vi "Get cif_manager_DestroyPluginLoaderResponse.vi"(8 "error in (no error)":errorcluster, 11 "gRPCid":T1) -> (0 "error out":errorcluster, 2 "package_templatemessage":T2, 3 "gRPCid out":T1)   [LabVIEW 2021, in "CIF_PluginLoader_server.lvlib"]
uses:
  CIF_PluginLoader_server.lvlib
  cif_manager_DestroyPluginLoaderResponse.ctl
  cif_common_Status.ctl
  <vilib>/gRPC/LabVIEW gRPC Library/Shared/grpcId.ctl
  cif_manager_DestroyPluginLoaderResponse_Flat.ctl
  cif_common_Status_Flat.ctl
  2ed25e12-861d-4677-8ead-ace2906b2041.vi
  <vilib>/gRPC/LabVIEW gRPC Library/Shared/TranslateGrpcError.vi
  FlatToRichcif_common_Status.vi
  <vilib>/gRPC/LabVIEW gRPC Library/Server API/Server/Get Server DLL Path.vi
  <vilib>/Utility/error.llb/Error Cluster From Error Code.vi
  <vilib>/gRPC/LabVIEW gRPC Library/grpc-lvsupport-release.lvlib
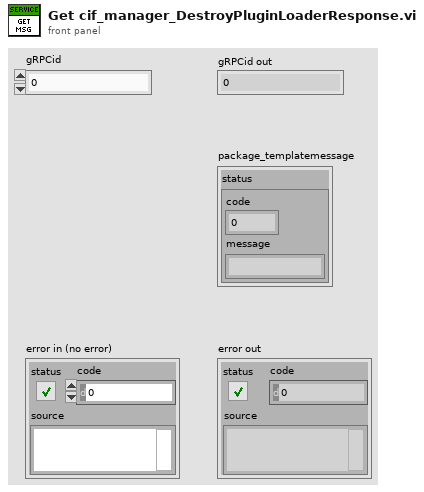
[diagram p1: front panel]
types:
  T1 = typedef "grpc-lvsupport-release.lvlib/grpcId.ctl" = u64
  T2 = typedef "CIF_PluginLoader_server.lvlib/cif_manager_DestroyPluginLoaderResponse.ctl" = cluster{"status":T3}
  T3 = typedef "CIF_PluginLoader_server.lvlib/cif_common_Status.ctl" = cluster{"code":i32, "message":string}
  T4 = typedef "CIF_PluginLoader_server.lvlib/cif_manager_DestroyPluginLoaderResponse_Flat.ctl" = cluster{"status":T5}
  T5 = typedef "CIF_PluginLoader_server.lvlib/cif_common_Status_Flat.ctl" = cluster{"code":i32, "message":string}
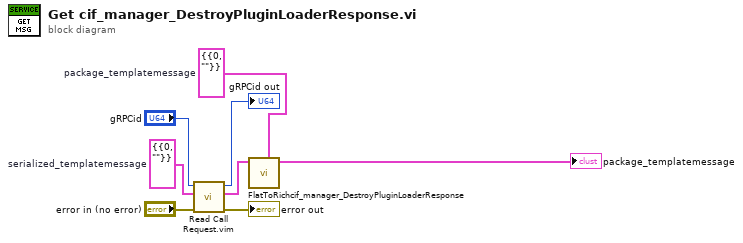
[diagram p0: block diagram]
diagram:
  w6 = T4 {"status"={"code"=0, "message"=""}}  # serialized_templatemessage
  w5 = T2 {"status"={"code"=0, "message"=""}}  # package_templatemessage
  n1 = call "Read Call Request.vim"("error in"="error in (no error)", "Request Type"=w6, "gRPCid in"="gRPCid") -> ("error out"=→"error out":errorcluster, "Request Data"=w4:T4, "gRPCid out"=→"gRPCid out":T1)  [unwired: 6 in]
  n2 = call "FlatToRichcif_manager_DestroyPluginLoaderResponse.vi"("OutputClusterType"=w5, "InputCluster"=w4) -> ("OutputCluster"=→"package_templatemessage":T2)  [unwired: 9 in]
